vi "Write Multiple Holding Registers.vi"(8 "error in (no error)":errorcluster, 9 "values":u16[](array[numeric]), 10 "address":u16, 11 "MODBUS in":refnum<class "PL Modbus Client.lvclass">) -> (0 "error out":errorcluster, 3 "MODBUS out":refnum<class "PL Modbus Client.lvclass">)   [LabVIEW 2015, in "PL Modbus Client.lvclass"]
doc: "Writes multiple holding register <B>values</B> starting at specified <B>address</B> (Modbus function code: <B>16</B>)."
uses:
  PL Modbus Client.lvclass
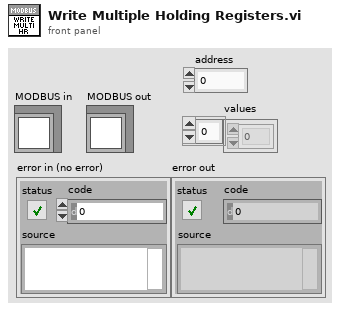
[diagram p1: front panel]
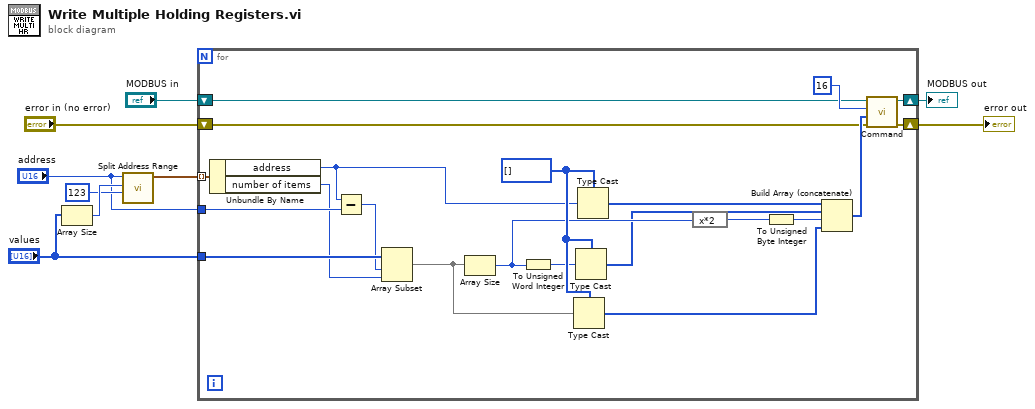
[diagram p0: block diagram]
diagram:
  n1 = Array Size(array="values") -> (size(s)=w7:i32)
  n2 = call "Split Address Range.vi"("max number of items"=u16 123, "number of items"=w7, "address"="address") -> ("addresses and numbers of items"=w5:cluster{"address":u16, "number of items":u16}[])  [unwired: 8 in]
  n3 = for {
    tunnel: "values" -> [w28]
    shift-right: [w10] -> w8
    shift-left: "MODBUS in" -> [w12]
    shift-right: [w13] -> w2
    shift-left: "error in (no error)" -> [w11]
    tunnel: w5 -> [w30] mode=indexing
    tunnel: "address" -> [w29]
    w25 = u8[] []
    n4 = Unbundle By Name(w30) -> ("address"=w15:u16, "number of items"=w26:u16)
    n5 = Subtract(x=w15, y=w29) -> (x-y=w27:u16)
    n6 = Array Subset(array=w28, index=w27, length=w26) -> (w14:u16[])
    n7 = Array Size(array=w14) -> (size(s)=w22:i32)
    n8 = To Unsigned Word Integer(number=w22) -> (unsigned 16bit integer=w20:u16)
    n9 = Type Cast(type=w25, x=w14) -> (*(type *) &x=w24:u8[])
    n10 = Type Cast(type=w25, x=w20) -> (*(type *) &x=w17:u8[])
    n11 = Type Cast(type=w25, x=w15) -> (*(type *) &x=w16:u8[])
    n12 = expression code="x*2"(w22) -> (w23:i32)
    n13 = To Unsigned Byte Integer(number=w23) -> (unsigned 8bit integer=w21:u8)
    n14 = Build Array (concatenate)(w16, w17, w21, w24) -> (w18:u8[])
    n15 = call "Command.vi"("error in (no error)"=w11, "data in"=w18, "function code"=u8 16 ("function"), "MODBUS in"=w12) -> ("error out"=w13:errorcluster, "MODBUS out"=w10:refnum<class "PL Modbus Client.lvclass">)  [unwired: 5 in, 1 out]
  }
  "MODBUS out" <- w8
  "error out" <- w2
